vi "CreateSensorChannelNames (SubVI).vi"(3 "channel name":string[](array[string]), 5 "sensor count (default: 14)":i32=14) -> (1 "channel names":string[](array[string]))   [LabVIEW 2017]
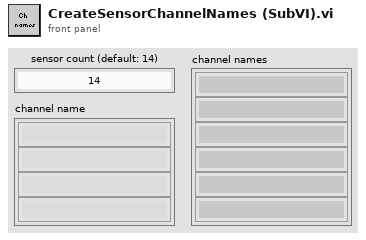
[diagram p1: front panel]
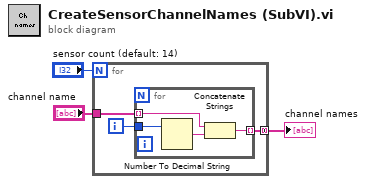
[diagram p0: block diagram]
diagram:
  n1 = for {
    N: "sensor count (default: 14)" -> [_]
    tunnel: "channel name" -> [w6]
    tunnel: [w4] -> w3 mode=concatenating
    i -> [w5]
    n2 = for {
      tunnel: w6 -> [w10] mode=indexing
      tunnel: w5 -> [w9]
      tunnel: [w7] -> w4 mode=indexing
      n3 = Number To Decimal String(number=w9) -> (decimal integer string=w8:string)  [unwired: 1 in]
      n4 = Concatenate Strings(w10, w8) -> (w7:string)
    }
  }
  "channel names" <- w3
